vi "总磷总氮操作日志.vi"(8 "错误输入（无错误）":errorcluster, 11 "data in":T1) -> (0 "错误输出":errorcluster)   [LabVIEW 2016, in "斯坦道氨氮.lvlib"]
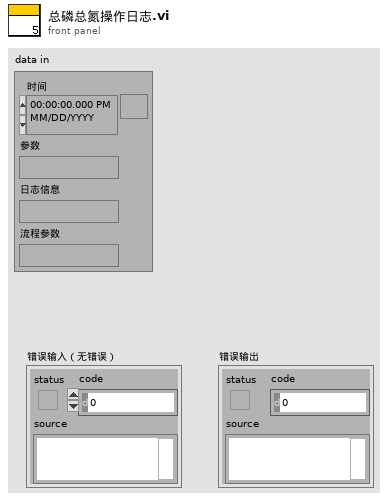
[diagram p1: front panel]
types:
  T1 = typedef "操作日志字段定义.ctl" = cluster{"时间":timestamp, "参数":string, "日志信息":string, "流程参数":string}
  T2 = typedef "数据库类型.ctl" = enum16{"Access", "SQLite"}
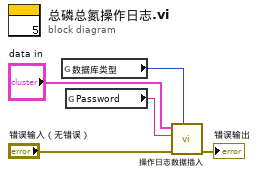
[diagram p0: block diagram]
diagram:
  n1 = global read "总磷总氮断电保存全局变量.vi" "数据库类型"() -> (w4:T2)
  n2 = global read "总磷总氮断电保存全局变量.vi" "Password"() -> (w1:string)
  n3 = call "操作日志数据插入.vi"("data"="data in", "Password"=w1, "错误输入（无错误）"="错误输入（无错误）", "数据库类型"=w4) -> ("错误输出"=→"错误输出":errorcluster)  [unwired: 6 in]
